vi "HumanGlobal.vi"() -> ()   [LabVIEW 2020]
panel:
  out "CurrentAction":string
  out "Reverse":bool
  out "StateChange":bool
  out "DPadLeft":bool
  out "DPadRight":bool
  out "DPadDown":bool
  out "DPadUp":bool
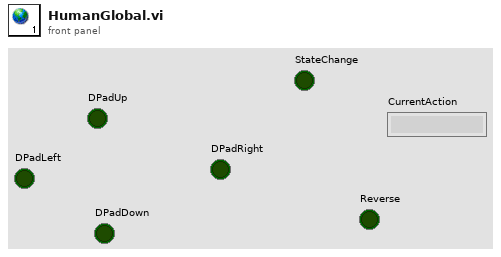
[diagram p1: front panel]
diagram:
